vi "remote.Get Property Enum Value Names.vi"(0 "SLSC Remote in":refnum<class "SLSC Interface.lvclass">, 5 "property":refnum<k21>, 11 "error in (no error)":errorcluster) -> (4 "SLSC Remote out":refnum<class "SLSC Interface.lvclass">, 6 "property out":refnum<k21>, 10 "Prop.Enum.ValueNames":string[](array[string]), 15 "error out":errorcluster)   [LabVIEW 2016, in "SLSC Interfaces.lvlib" / "SLSC Interface.lvclass"]
uses:
  SLSC Interface Class/SLSC Interface.lvclass
  <vilib>/NI/NI JSONRPC Server Framework/Classes/Server/JSONRPC Server.lvclass
  <vilib>/httpClient/LabVIEWHTTPClient.lvlib
  <vilib>/httpClient/POSTBuffer.vi
  <vilib>/NI/JSON Support for LabVIEW/JSON Data Classes/JSON Helper/JSON Helper.lvclass
  <vilib>/NI/JSON Support for LabVIEW/JSON Data Classes/JSON Object/JSON Object.lvclass
  <vilib>/NI/JSON Support for LabVIEW/JSON Data Classes/JSON Object/Get Value (Array).vi
  <vilib>/NI/JSON Support for LabVIEW/JSON Data Classes/JSON Helper/To More Specific Type (Object).vi
  <vilib>/NI/JSON Support for LabVIEW/JSON Data Classes/JSON Array/JSON Array.lvclass
  <vilib>/NI/JSON Support for LabVIEW/JSON Data Classes/JSON Array/Index Array (String Value).vi
  <vilib>/NI/JSON Support for LabVIEW/JSON Data Classes/JSON Object/New JSON Object (Empty).vi
  <vilib>/NI/JSON Support for LabVIEW/JSON Data Classes/JSON Object/Insert Key Value Pair (Single String).vi
  <vilib>/NI/NI JSONRPC Server Framework/Classes/Server/Format Client Request (Auto-Increment).vi
  <vilib>/NI/NI JSONRPC Server Framework/Classes/Server/Parse Response (JSON).vi
  C:/Program Files (x86)/National Instruments/LabVIEW 2016/vi.lib/NI/JSON Support for LabVIEW/JSON Data Classes/JSON Structured Type/JSON Structure.lvclass
  C:/Program Files (x86)/National Instruments/LabVIEW 2016/vi.lib/NI/JSON Support for LabVIEW/JSON Data Classes/JSON Datatype/JSON Null.lvclass
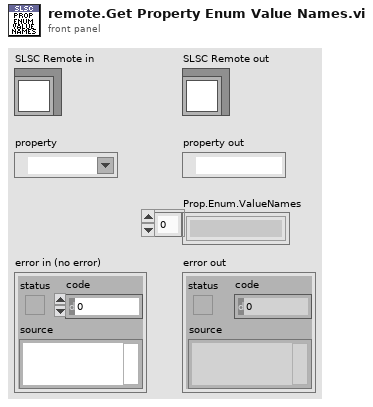
[diagram p1: front panel]
types:
  T1 = typedef "LabVIEWHTTPClient.lvlib/ClientHandle.ctl" = refnum<k1>
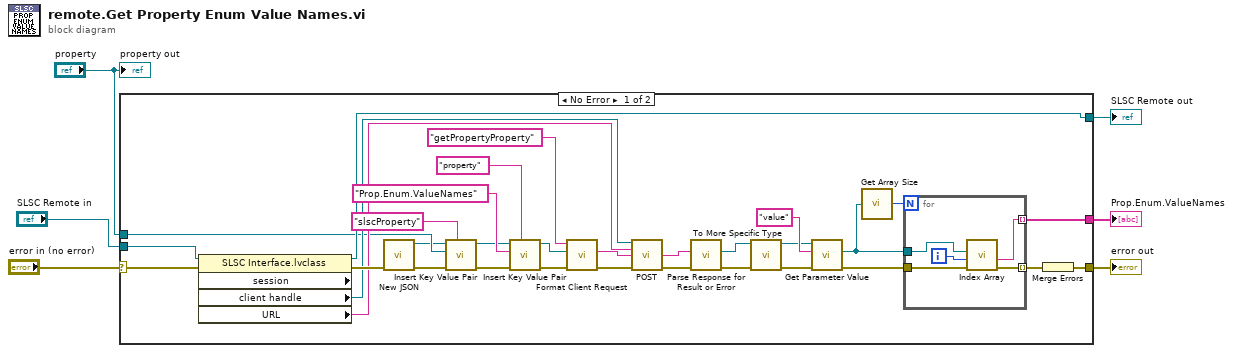
[diagram p0: block diagram]
diagram:
  n1 = case shown="No Error" "error in (no error)" {
    selector: "error in (no error)" -> [w36 w44]
    tunnel: "SLSC Remote in" -> [w38 w45]
    tunnel: [w37 w45] -> w4
    tunnel: [w14 w44] -> w1
    tunnel: [w15 _] -> w2
    tunnel: "property" -> [w13 _]
    frame No Error {
      n2 = property class="SLSC Interface.lvclass" props=["session", "client handle", "URL"](reference=w38, error in=w36) -> (reference out=w37:refnum<class "SLSC Interface.lvclass">, error out=w35:errorcluster, "client handle"=w31:T1, "URL"=w30:string)  [unwired: 1 out]
      n3 = call-poly <vilib>:"New JSON.vi"("error in (no error)"=w35) -> ("error out"=w34:errorcluster, "JSON Object out"=w11:refnum<class "JSON Object.lvclass">)  [unwired: 9 in]
      n4 = call-poly <vilib>:"Insert Key Value Pair.vi"("key"="slscProperty" ("Name"), "error in (no error)"=w34, "value"=w13, "JSON Object in"=w11) -> ("error out"=w24:errorcluster, "JSON Object out"=w10:refnum<class "JSON Object.lvclass">)  [unwired: 5 in, 1 out]
      n5 = call-poly <vilib>:"Insert Key Value Pair.vi"("key"="property" ("Name"), "error in (no error)"=w24, "value"="Prop.Enum.ValueNames" ("String"), "JSON Object in"=w10) -> ("error out"=w25:errorcluster, "JSON Object out"=w26:refnum<class "JSON Object.lvclass">)  [unwired: 5 in, 1 out]
      n6 = call-poly <vilib>:"Format Client Request.vi"("error in (no error)"=w25, "JSON in"=w26, "method"="getPropertyProperty") -> ("error out"=w29:errorcluster, "Request String"=w32:string)  [unwired: 7 in]
      n7 = call-poly <vilib>:"POST.vi"("client handle"=w31, "url"=w30, "buffer"=w32, "error in (no error)"=w29) -> ("body"=w28:string, "error out"=w27:errorcluster)  [unwired: 8 in, 2 out]
      n8 = call-poly <vilib>:"Parse Response for Result or Error.vi"("error in"=w27, "Response String In"=w28) -> ("error out"=w7:errorcluster, "JSON out"=w16:refnum<class "JSON Null.lvclass">)  [unwired: 7 in, 1 out]
      n9 = call-poly <vilib>:"To More Specific Type.vi"("error in (no error)"=w7, "JSON Datatype in"=w16) -> ("error out"=w22:errorcluster, "JSON Datatype out"=w21:refnum<class "JSON Object.lvclass">)  [unwired: 8 in]
      n10 = call-poly <vilib>:"Get Parameter Value.vi"("error in (no error)"=w22, "key"="value" ("Parameter Name"), "JSON Object in"=w21) -> ("error out"=w18:errorcluster, "value"=w19:refnum<class "JSON Array.lvclass">)  [unwired: 7 in]
      n11 = call <vilib>:"Get Array Size.vi"("JSON Array in"=w19) -> ("size(s)"=w20:i32)
      n12 = for {
        N: w20 -> [_]
        tunnel: w19 -> [w42]
        tunnel: w18 -> [w41]
        tunnel: [w40] -> w17 mode=indexing
        tunnel: [w39] -> w15 mode=indexing
        i -> [w43]
        n13 = call-poly <vilib>:"Index Array.vi"("error in (no error)"=w41, "index"=w43, "JSON Array in"=w42) -> ("error out"=w40:errorcluster, "String"=w39:string)  [unwired: 7 in]
      }
      n14 = Merge Errors(w17) -> (w14:errorcluster)
    }
    frame Error {
    }
  }
  "error out" <- w1
  "SLSC Remote out" <- w4
  "Prop.Enum.ValueNames" <- w2
  "property out" <- "property"
